vi "Get google_protobuf_EnumValue.vi"(8 "error in (no error)":errorcluster, 11 "gRPCid":T1) -> (0 "error out":errorcluster, 2 "package_templatemessage":T2, 3 "gRPCid out":T1)   [LabVIEW 2021, in "ni.measurementlink.measurement.v2.api.lvlib"]
uses:
  ni.measurementlink.measurement.v2.api.lvlib
  google_protobuf_EnumValue.ctl
  google_protobuf_Option.ctl
  google_protobuf_Any.ctl
  <vilib>/gRPC/LabVIEW gRPC Library/Shared/grpcId.ctl
  google_protobuf_EnumValue_Flat.ctl
  google_protobuf_Option_Flat.ctl
  google_protobuf_Any_Flat.ctl
  2ed25e12-861d-4677-8ead-ace2906b2041.vi
  <vilib>/gRPC/LabVIEW gRPC Library/Shared/TranslateGrpcError.vi
  FlatToRichgoogle_protobuf_Option.vi
  FlatToRichgoogle_protobuf_Any.vi
  <vilib>/gRPC/LabVIEW gRPC Library/Server API/Server/Get Server DLL Path.vi
  <vilib>/Utility/error.llb/Error Cluster From Error Code.vi
  <vilib>/gRPC/LabVIEW gRPC Library/grpc-lvsupport-release.lvlib
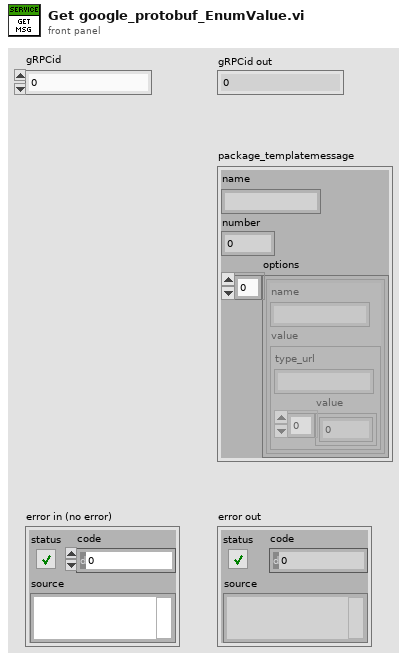
[diagram p1: front panel]
types:
  T1 = typedef "grpc-lvsupport-release.lvlib/grpcId.ctl" = u64
  T2 = typedef "ni.measurementlink.measurement.v2.api.lvlib/google_protobuf_EnumValue.ctl" = cluster{"name":string, "number":i32, "options":T3[]}
  T3 = typedef "ni.measurementlink.measurement.v2.api.lvlib/google_protobuf_Option.ctl" = cluster{"name":string, "value":T4}
  T4 = typedef "ni.measurementlink.measurement.v2.api.lvlib/google_protobuf_Any.ctl" = cluster{"type_url":string, "value":u8[]}
  T5 = typedef "ni.measurementlink.measurement.v2.api.lvlib/google_protobuf_EnumValue_Flat.ctl" = cluster{"name":string, "number":i32, "options":T6[]}
  T6 = typedef "ni.measurementlink.measurement.v2.api.lvlib/google_protobuf_Option_Flat.ctl" = cluster{"name":string, "value":T7}
  T7 = typedef "ni.measurementlink.measurement.v2.api.lvlib/google_protobuf_Any_Flat.ctl" = cluster{"type_url":string, "value":u8[]}
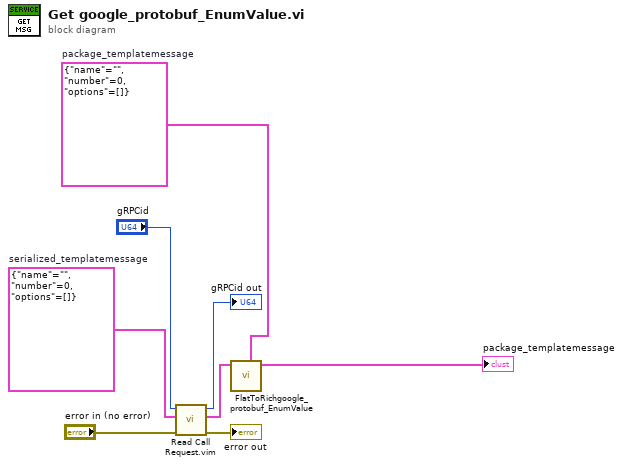
[diagram p0: block diagram]
diagram:
  w6 = T5 {"name"="", "number"=0, "options"=[]}  # serialized_templatemessage
  w5 = T2 {"name"="", "number"=0, "options"=[]}  # package_templatemessage
  n1 = call "Read Call Request.vim"("error in"="error in (no error)", "Request Type"=w6, "gRPCid in"="gRPCid") -> ("error out"=→"error out":errorcluster, "Request Data"=w4:T5, "gRPCid out"=→"gRPCid out":T1)  [unwired: 6 in]
  n2 = call "FlatToRichgoogle_protobuf_EnumValue.vi"("OutputClusterType"=w5, "InputCluster"=w4) -> ("OutputCluster"=→"package_templatemessage":T2)  [unwired: 9 in]
